vi "Host View Process.vi"(8 "error in (no error)":errorcluster, 11 "View Model":T8) -> (0 "error out":errorcluster)   [LabVIEW 2017]
doc: "PC Host based UI component for interaction with user"
uses:
  View Model/Controls/View Model.ctl
  View Model/Controls/Shared Model.ctl
  Error Handler/Controls/Error Model.ctl
  Error Handler/Controls/Error Event.ctl
  Error Handler/Controls/Error Type.ctl
  Controller/Controls/Controller Model.ctl
  Controller/Controls/Controller Event.ctl
  Controller/Controls/Controller Command.ctl
  Controller/Controls/Controller Overhead.ctl
  Real-Time/RT Status.ctl
  Real-Time/RT Loop Status.ctl
  Controller/Controls/Controller NStream.ctl
  Controller/Controls/Controller DAQ Data.ctl
  TDMS Logger/Controls/TDMS Model.ctl
  TDMS Logger/Controls/TDMS Event.ctl
  TDMS Logger/Controls/TDMS Command.ctl
  TDMS Logger/Controls/TDMS Overhead.ctl
  TDMS Logger/Controls/TDMS ChanProperties.ctl
  Controls/AIMV_GUI_Cluster.ctl
  Controls/AIMC_GUI_Cluster.ctl
  Controls/AOM_GUI_Cluster.ctl
  Controls/Discrete_GUI_Cluster.ctl
  Controls/GUI Referencies.ctl
  <resource>/objmgr/ni.dex.rc
panel:
  out "FileSize":i32
  out "Use TDMS?":bool
  in  "TDMS Close":bool
  in  "TDMS Save":bool
  in  "TDMS Create":bool
  in  "DOM7 Array":T1[](array[typedef])
  in  "DIM4 Array":T1[](array[typedef])
  out "DAQ Data":T2
  in  "DAQ read":bool
  in  "DAQ write":bool
  out "NStream.exist?":bool
  out "Available":i32
  out "size(s)":i32[](array[numeric])
  in  "NW Start/Stop":bool
  in  "DOM6 Array":T1[](array[typedef])
  in  "DIM3 Array":T1[](array[typedef])
  in  "AOM9 Array":T3[](array[typedef]) {"Ch.value" min=-10.0 max=20.0 step=1.0 format="%.3g"}
  in  "AIMC Array":T4[](array[typedef]) {"Ch.value" min=0.0 max=20.1 step=1.0 format="%.3g"}
  in  "AIM2 Array":T5[](array[typedef]) {"Ch.value" min=-10.0 max=10.0 step=1.0 format="%05.3f"}
  out "RT Status":T6 {"Status NPL"."Duration, us" format="%0.2f"; "Status TCL2"."Duration, us" format="%0.2f"; "Status TCL1"."Duration, us" format="%0.2f"}
  in  "Stop RT":bool
  out "Blink1":bool
  in  "Stop App":bool
  in  "Init":bool
  # "DAQ data"
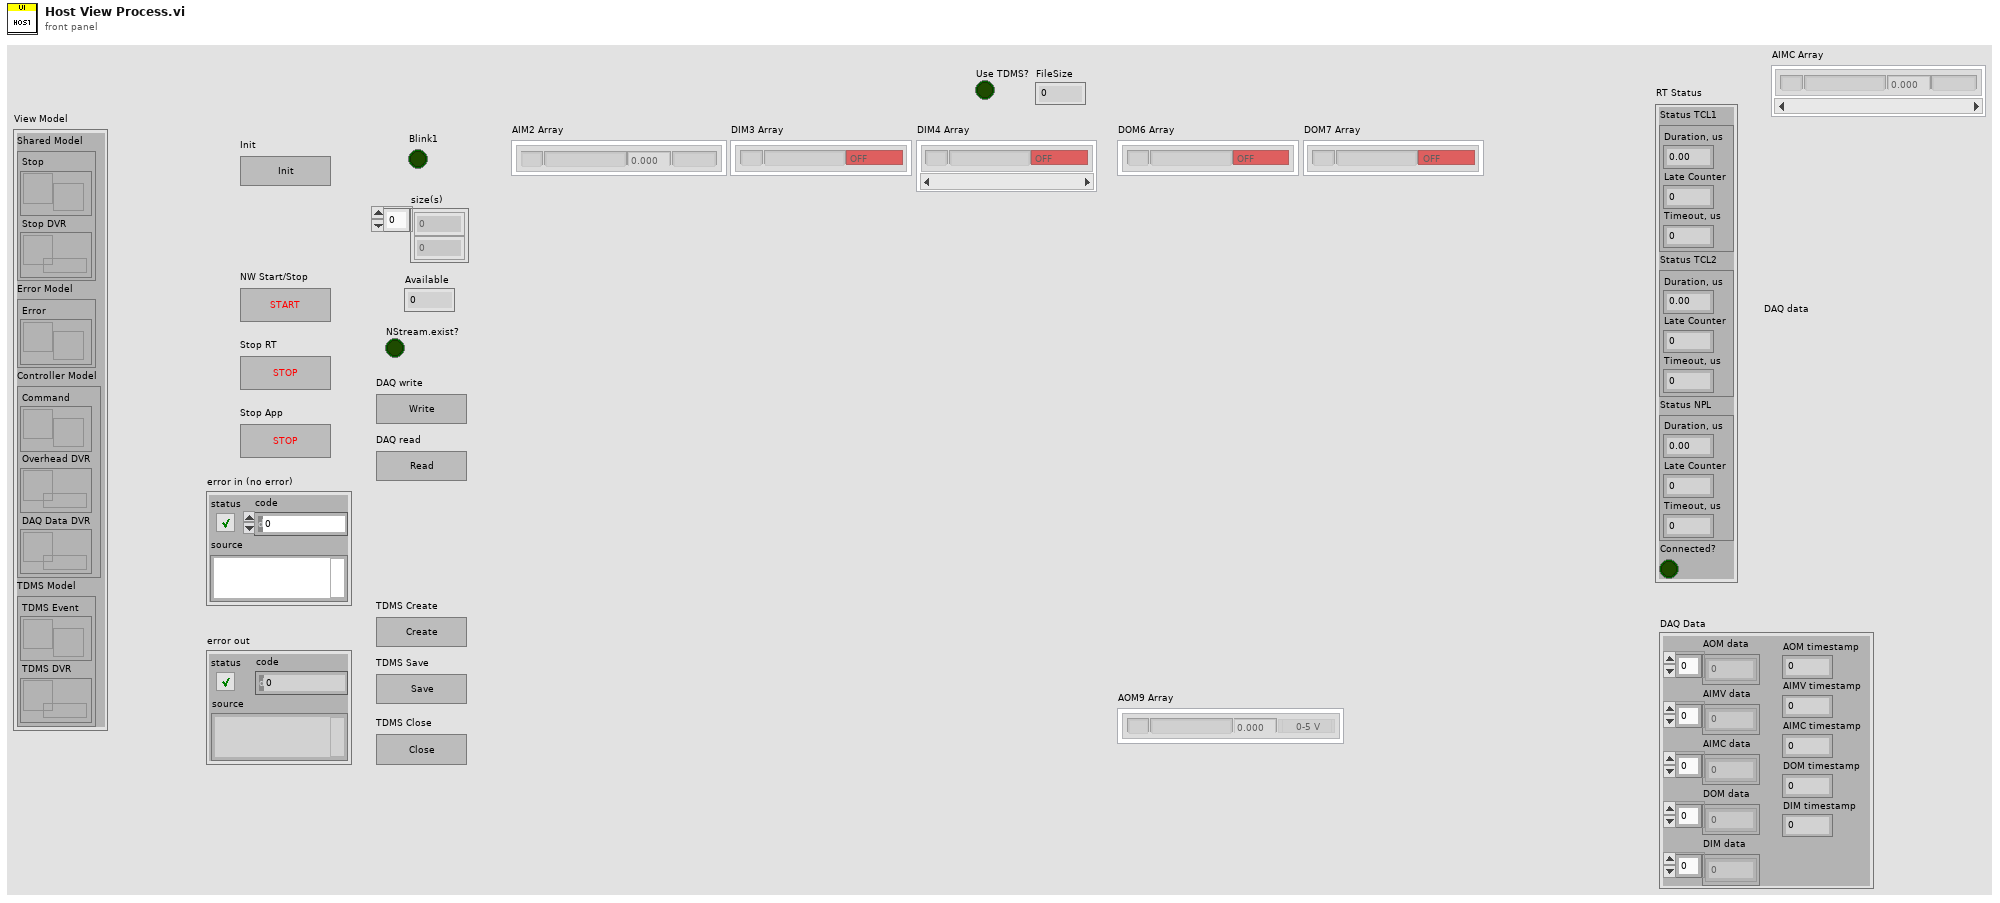
[diagram p1: front panel]
types:
  T1 = typedef "Discrete_GUI_Cluster.ctl" = cluster{"Ch.name":string, "Ch.state":bool, "Num":string}
  T2 = typedef "Controller DAQ Data.ctl" = cluster{"AOM data":dbl[], "AIMV data":dbl[], "AIMC data":dbl[], "DOM data":dbl[], "DIM data":dbl[], "AOM timestamp":dbl, "AIMV timestamp":dbl, "AIMC timestamp":dbl, "DOM timestamp":dbl, "DIM timestamp":dbl}
  T3 = typedef "AOM_GUI_Cluster.ctl" = cluster{"Ch.name":string, "Ch.value":dbl, "Ch.mode":enum16{"0-5 V", "+/-10 V", "0-5 mA", "4-20 mA"}, "Num":string}
  T4 = typedef "AIMC_GUI_Cluster.ctl" = cluster{"Ch.name":string, "Ch.value":dbl, "Ch.range":string, "Num":string}
  T5 = typedef "AIMV_GUI_Cluster.ctl" = cluster{"Ch.name":string, "Ch.value":dbl, "Ch.range":string, "Num":string}
  T6 = typedef "RT Status.ctl" = cluster{"Status TCL1":T7, "Status TCL2":T7, "Status NPL":T7, "Connected?":bool}
  T7 = typedef "RT Loop Status.ctl" = cluster{"Duration, us":dbl, "Late Counter":i32, "Timeout, us":u32}
  T8 = typedef "View Model.ctl" = cluster{"Shared Model":T9, "Error Model":T10, "Controller Model":T11, "TDMS Model":T12}
  T9 = typedef "Shared Model.ctl" = cluster{"Stop":refnum<user-event>, "Stop DVR":refnum<data-value>}
  T10 = typedef "Error Model.ctl" = cluster{"Error":refnum<user-event>}
  T11 = typedef "Controller Model.ctl" = cluster{"Command":refnum<user-event>, "Overhead DVR":refnum<data-value>, "DAQ Data DVR":refnum<data-value>}
  T12 = typedef "TDMS Model.ctl" = cluster{"TDMS Event":refnum<user-event>, "TDMS DVR":refnum<data-value>}
  T13 = typedef "GUI Referencies.ctl" = cluster{"This VI":refnum<vi>, "This App":refnum<vi>, "DIM3":refnum<vi>, "DIM4":refnum<vi>, "DOM6":refnum<vi>, "DOM7":refnum<vi>, "AOM9":refnum<vi>, "AIM2":refnum<vi>, "AIMC":refnum<vi>}
  T14 = typedef "Controller Command.ctl" = enum16{"Idle", "Init", "Stop App", "Stop RT", "NStream Create", "NStream Begin", "NStream End", "NStream Close", "DAQ Data Read", "DAQ Data Write", "TDMS Restart"}
  T15 = typedef "Error Type.ctl" = enum16{"Minor", "Critical"}
  T16 = typedef "TDMS Command.ctl" = enum16{"Idle", "Create File", "Save Data", "Close Fire"}
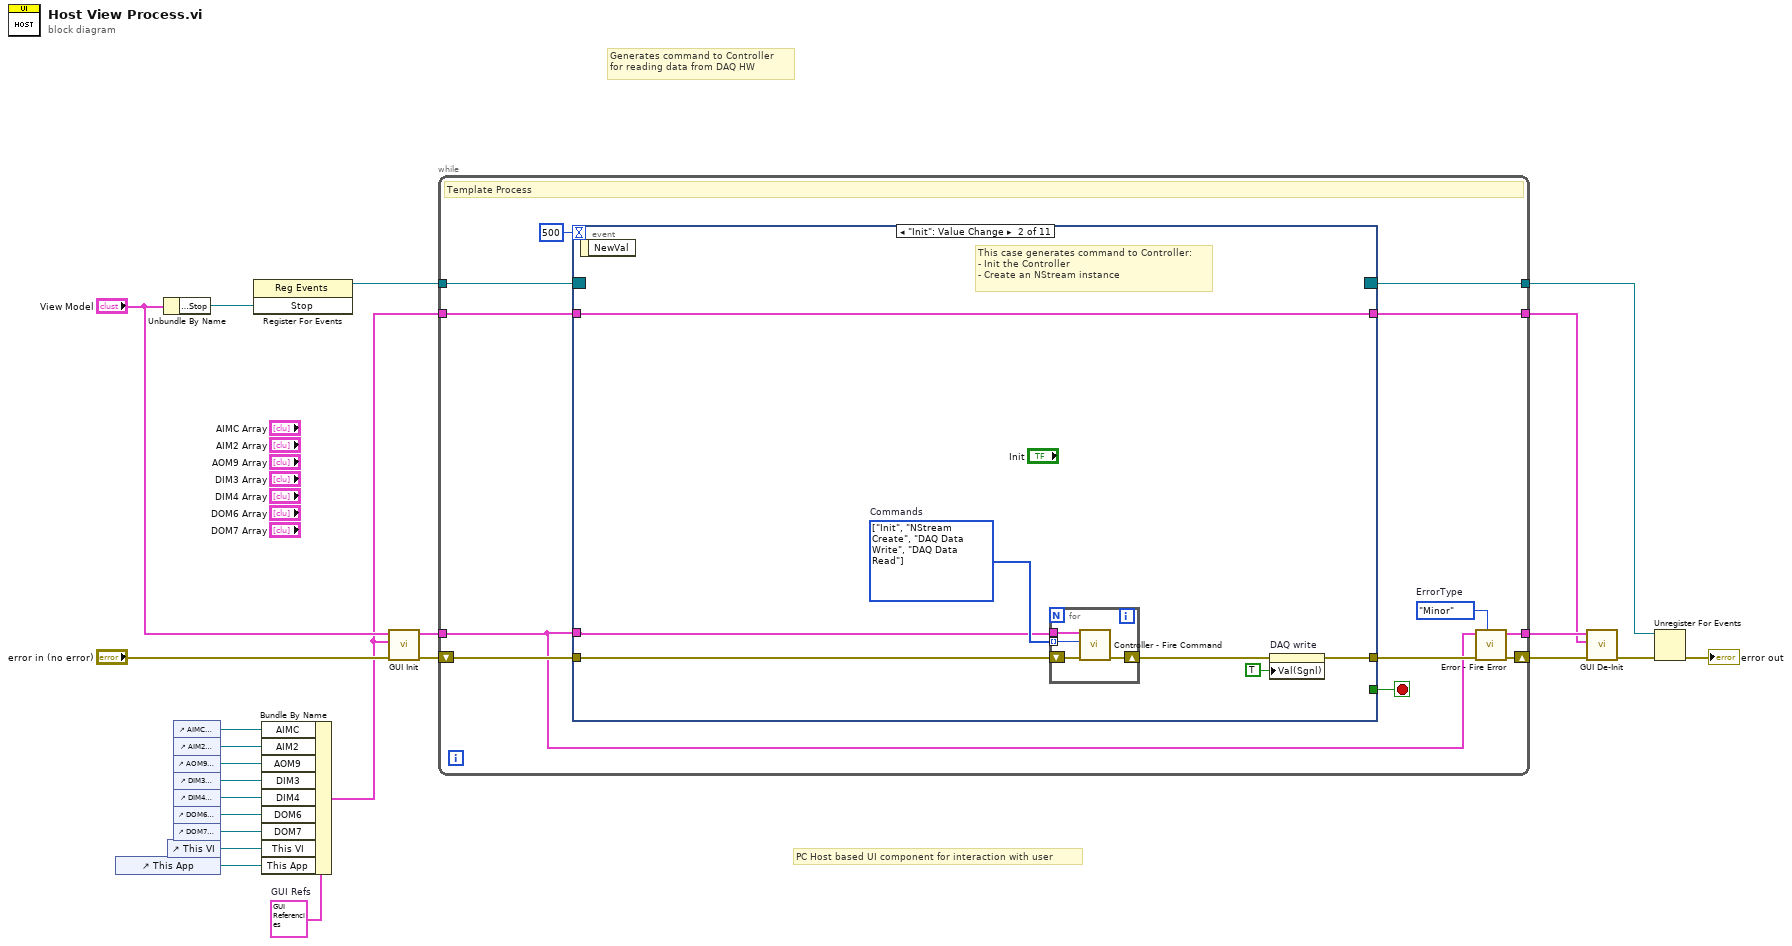
[diagram p0: block diagram]
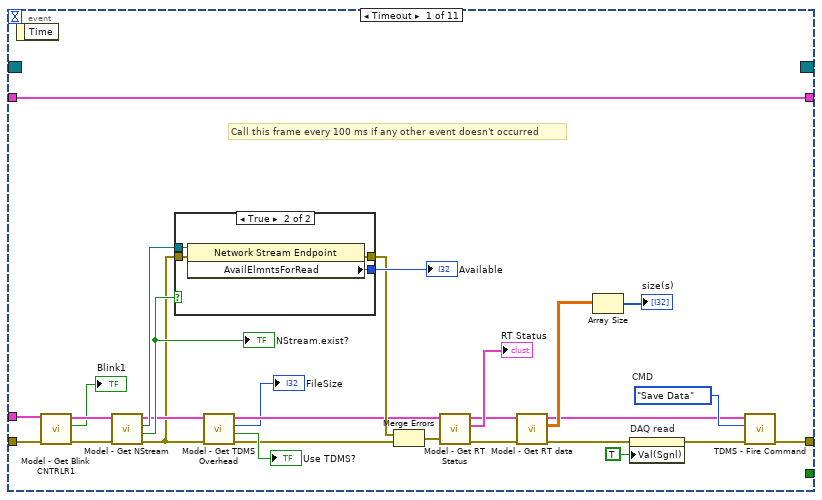
[diagram p2: hidden frame]
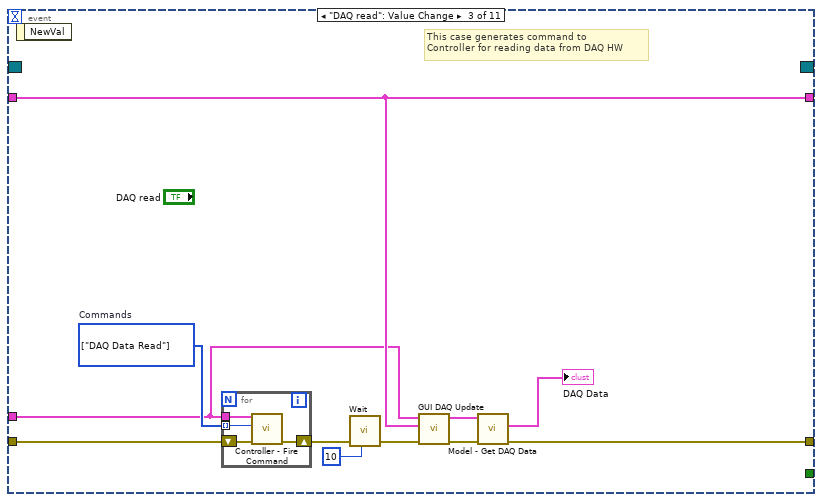
[diagram p4: hidden frame]
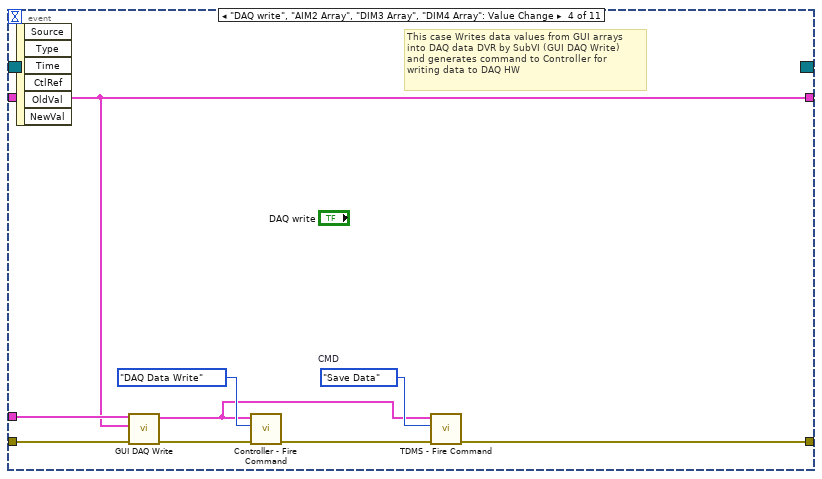
[diagram p5: hidden frame]
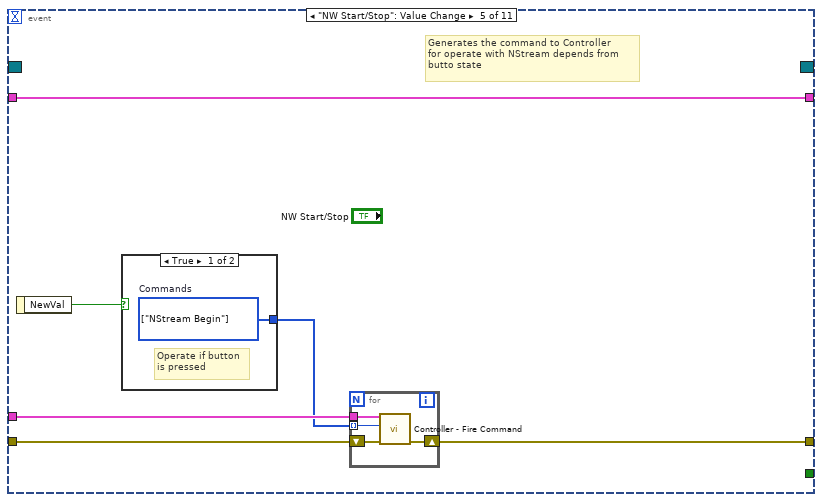
[diagram p6: hidden frame]
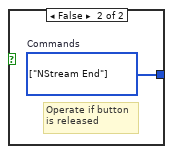
[diagram p7: hidden frame]
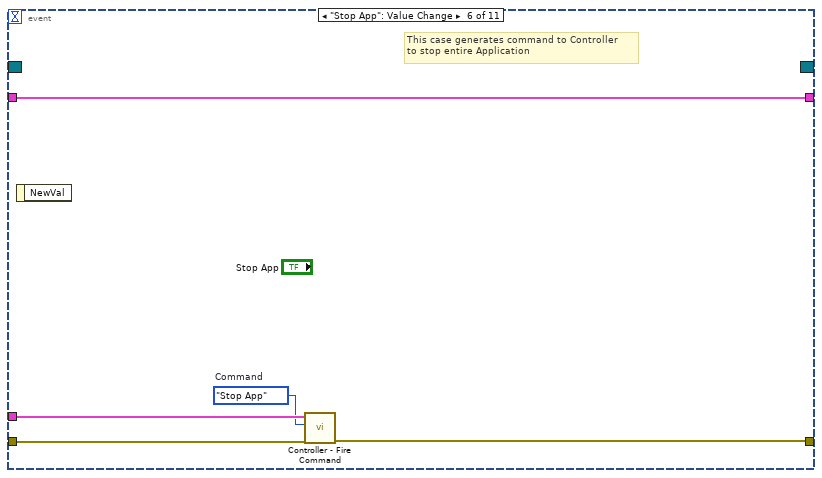
[diagram p8: hidden frame]
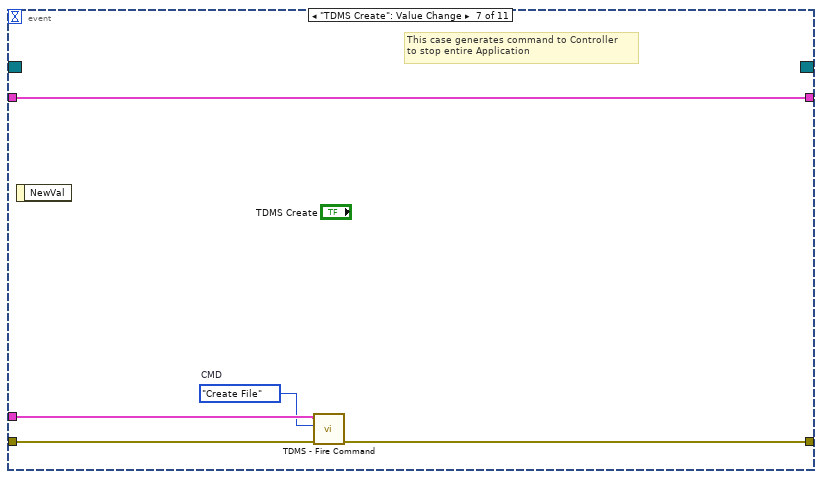
[diagram p9: hidden frame]
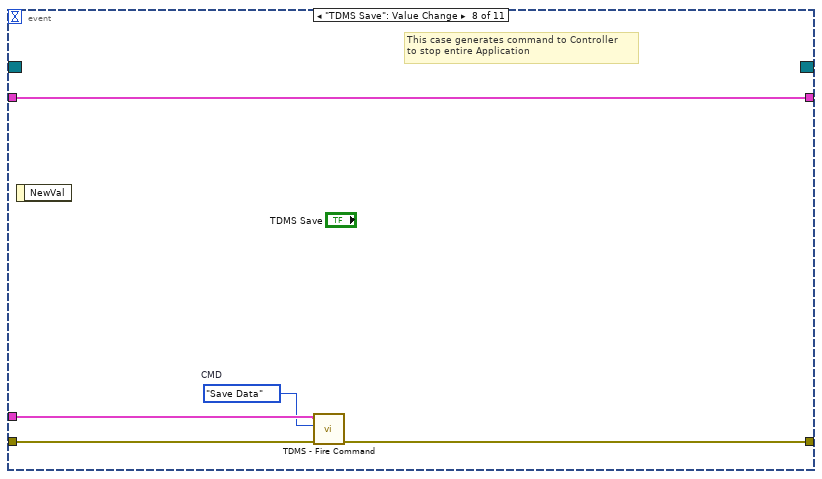
[diagram p10: hidden frame]
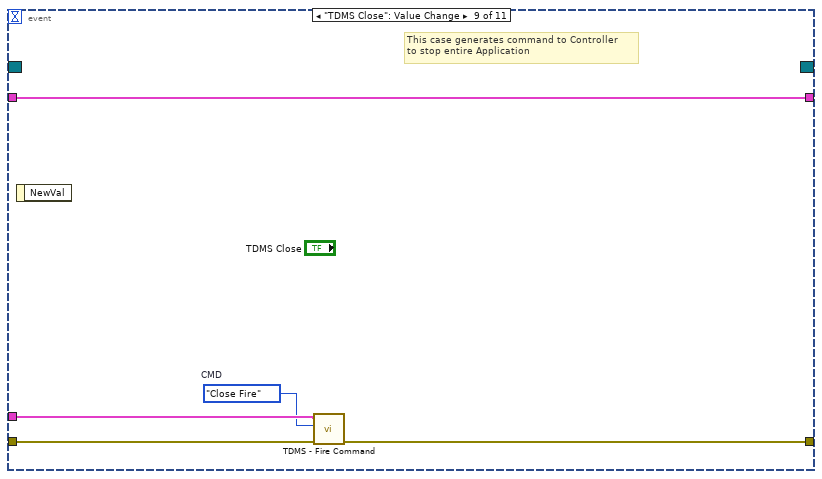
[diagram p11: hidden frame]
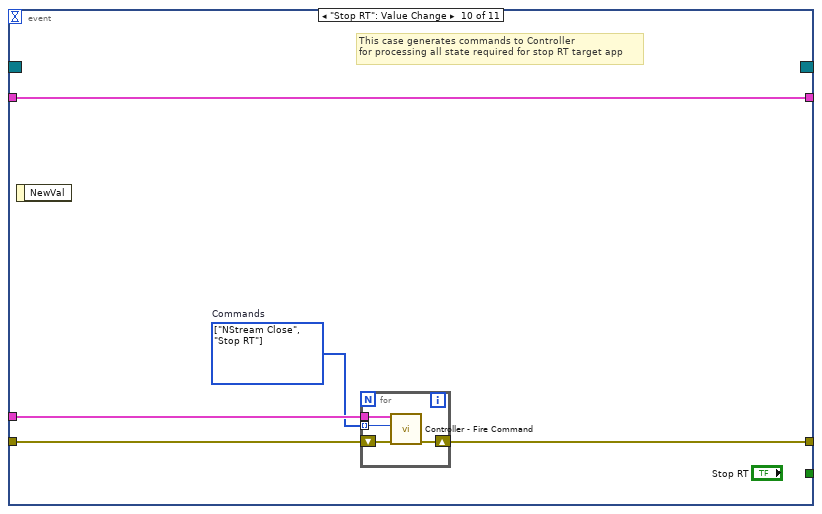
[diagram p12: hidden frame]
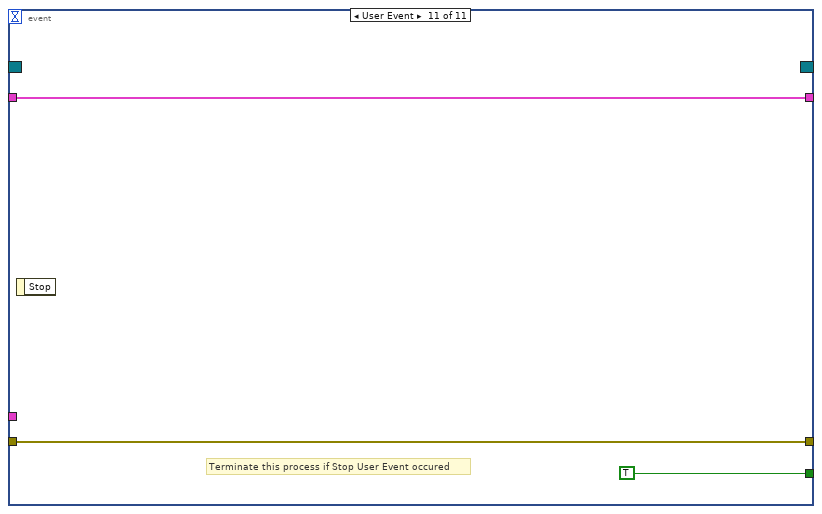
[diagram p13: hidden frame]
diagram:
  w12 = T13 {"This VI"=refnum, "This App"=refnum, "DIM3"=refnum, "DIM4"=refnum, "DOM6"=refnum, "DOM7"=refnum, "AOM9"=refnum, "AIM2"=refnum, "AIMC"=refnum}  # GUI Refs
  # "Generates command to Controller \nfor reading data from DAQ HW"
  # "PC Host based UI component for interaction with user"
  n1 = control-ref of="This App"() -> (w11:refnum<vi>)
  n2 = Unbundle By Name("View Model") -> ("Shared Model.Stop"=w23:refnum<user-event>)
  n3 = control-ref of="This VI"() -> (w10:refnum<vi>)
  n4 = control-ref of="AIMC Array"() -> (w1:refnum<vi>)
  n5 = control-ref of="AIM2 Array"() -> (w4:refnum<vi>)
  n6 = control-ref of="AOM9 Array"() -> (w3:refnum<vi>)
  n7 = control-ref of="DIM3 Array"() -> (w2:refnum<vi>)
  n8 = control-ref of="DIM4 Array"() -> (w5:refnum<vi>)
  n9 = control-ref of="DOM6 Array"() -> (w6:refnum<vi>)
  n10 = control-ref of="DOM7 Array"() -> (w7:refnum<vi>)
  n11 = register-events(w23) -> (reference out=w22:refnum<event-registration>)  [unwired: 2 in, 1 out]
  n12 = Bundle By Name(cluster=w12, "AIMC"=w1, "AIM2"=w4, "AOM9"=w3, "DIM3"=w2, "DIM4"=w5, "DOM6"=w6, "DOM7"=w7, "This VI"=w10, "This App"=w11) -> (w9:T13)
  n13 = call "GUI Init.vi"("error in (no error)"="error in (no error)", "GUI Refs"=w9, "View Model"="View Model") -> ("error out"=w18:errorcluster, "View Model"=w16:T8)  [unwired: 7 in]
  n14 = while {
    tunnel: w22 -> [w33]
    shift-right: [w29] -> w15
    shift-left: w18 -> [w35]
    tunnel: w16 -> [w28]
    tunnel: [w32] -> w21
    tunnel: [w27] -> w14
    tunnel: w9 -> [w25]
    tunnel: [w24] -> w8
    stop <- w31 stop-if-true
    w26 = Error_Type."Minor"  # ErrorType
    # "Template Process"
    n15 = event shown="[1] \"Init\": Value Change" {
      selector: w33 -> [_ _ _ _ _ _ _ _ _ _ _]
      dyn-events: [_ _ _ _ _ _ _ _ _ _ _] -> w32
      timeout: 500 -> [_ _ _ _ _ _ _ _ _ _ _]
      tunnel: w35 -> [w63 w69 w90 w103 w109 w120 w124 w129 w134 w140 w147]
      tunnel: w28 -> [w62 w70 w81 w102 w108 w119 w122 w127 w132 w139 _]
      tunnel: [w46 w72 w83 w96 w107 w118 w123 w128 w133 w138 w147] -> w30
      tunnel: [_ _ _ _ _ _ _ _ _ _ TRUE] -> w31
      tunnel: w25 -> [w51 w74 w82 w101 w104 w116 w125 w130 w135 w136 w145]
      tunnel: [w51 w74 w82 w101 w104 w116 w125 w130 w135 w136 w145] -> w24
      event Timeout {
        w48 = TDMS_Command."Save Data"  # CMD
        # "Call this frame every 100 ms if any other event doesn't occurred"
        n16 = event-data() -> ()  [unwired: 1 in, 1 out]
        n17 = call "Model - Get Blink CNTRLR1.vi"("error in (no error)"=w63, "View Model"=w62) -> ("error out"=w55:errorcluster, "BlinkC1"=→"Blink1":bool, "View Model"=w56:T8)  [unwired: 7 in]
        n18 = call "Model - Get NStream.vi"("error in (no error)"=w55, "View Model"=w56) -> ("error out"=w44:errorcluster, "NStream.exist?"=w52:bool, "NStream.Endpoint"=w54:refnum<k21>, "View Model"=w45:T8)  [unwired: 6 in]
        "NStream.exist?" <- w52
        n19 = case shown="True" w52 {
          tunnel: w44 -> [w64 w68]
          tunnel: w54 -> [_ w67]
          tunnel: [w64 w66] -> w49
          tunnel: [_ w65] -> w53
          frame False {
          }
          frame True {
            n20 = property class="Network Stream Endpoint"(reference=w67, error in=w68) -> (error out=w66:errorcluster, "AvailElmntsForRead"=w65:i32)  [unwired: 1 out]
          }
        }
        "Available" <- w53
        n21 = call "Model - Get TDMS Overhead.vi"("error in (no error)"=w44, "View Model"=w45) -> ("error out"=w40:errorcluster, "Use TDMS?"=→"Use TDMS?":bool, "FileSize"=→"FileSize":i32, "View Model"=w43:T8)  [unwired: 4 in, 2 out]
        n22 = Merge Errors(w49, w40) -> (w50:errorcluster)
        n23 = call "Model - Get RT Status.vi"("error in (no error)"=w50, "View Model"=w43) -> ("error out"=w60:errorcluster, "RT Status"=→"RT Status":T6, "View Model"=w59:T8)  [unwired: 7 in]
        n24 = call "Model - Get RT data.vi"("error in (no error)"=w60, "View Model"=w59) -> ("error out"=w39:errorcluster, "RT data"=w58:dbl[][], "View Model"=w47:T8)  [unwired: 7 in]
        n25 = Array Size(array=w58) -> (size(s)=→"size(s)":i32[])
        n26 = property on="DAQ read" class="Bool (strict)"(error in=w39, "Val(Sgnl)"=TRUE ("Value (Signaling)")) -> (error out=w38:errorcluster)  [unwired: 1 in, 1 out]
        n27 = call "TDMS - Fire Command.vi"("error in (no error)"=w38, "CMD"=w48, "View Model"=w47) -> ("error out"=w46:errorcluster)  [unwired: 8 in]
      }
      event "Init": Value Change {
        w75 = T14[] [enum."Init", enum."NStream Create", enum."DAQ Data Write", enum."DAQ Data Read"] items=["Idle", "Init", "Stop App", "Stop RT", "NStream Create", "NStream Begin", "NStream End", "NStream Close", "DAQ Data Read", "DAQ Data Write", "TDMS Restart"]  # Commands
        # "This case generates command to Controller:\n- Init the Controller\n- Create an NStream instance"
        n28 = event-data() -> ()  [unwired: 1 in, 1 out]
        n29 = for {
          tunnel: w70 -> [w78]
          shift-right: [w77] -> w73
          shift-left: w69 -> [w79]
          tunnel: w75 -> [w76] mode=indexing
          n30 = call "Controller - Fire Command.vi"("error in (no error)"=w79, "CMD"=w76, "View Model"=w78) -> ("error out"=w77:errorcluster)  [unwired: 8 in]
        }
        n31 = property on="DAQ write" class="Bool (strict)"(error in=w73, "Val(Sgnl)"=TRUE ("Value (Signaling)")) -> (error out=w72:errorcluster)  [unwired: 1 in, 1 out]
      }
      event "DAQ read": Value Change {
        w89 = T14[] [enum."DAQ Data Read"] items=["Idle", "Init", "Stop App", "Stop RT", "NStream Create", "NStream Begin", "NStream End", "NStream Close", "DAQ Data Read", "DAQ Data Write", "TDMS Restart"]  # Commands
        # "This case generates command to \nController for reading data from DAQ HW"
        n32 = event-data() -> ()  [unwired: 1 in, 1 out]
        n33 = for {
          tunnel: w81 -> [w93]
          shift-right: [w92] -> w88
          shift-left: w90 -> [w94]
          tunnel: w89 -> [w91] mode=indexing
          n34 = call "Controller - Fire Command.vi"("error in (no error)"=w94, "CMD"=w91, "View Model"=w93) -> ("error out"=w92:errorcluster)  [unwired: 8 in]
        }
        n35 = call "Wait.vi"("error in (no error)"=w88, "wait, ms"=u32 10) -> ("error out"=w84:errorcluster)  [unwired: 7 in]
        n36 = call "GUI DAQ Update.vi"("error in (no error)"=w84, "GUI Refs"=w82, "View Model"=w81) -> ("error out"=w86:errorcluster, "View Model"=w85:T8)  [unwired: 7 in]
        n37 = call "Model - Get DAQ Data.vi"("error in (no error)"=w86, "View Model"=w85) -> ("error out"=w83:errorcluster, "DAQ Data"=→"DAQ Data":T2)  [unwired: 7 in, 1 out]
      }
      event "DAQ write", "AIM2 Array", "DIM3 Array", "DIM4 Array": Value Change {
        w98 = TDMS_Command."Save Data"  # CMD
        # "This case Writes data values from GUI arrays\ninto DAQ data DVR by SubVI (GUI DAQ Write)\nand generates command to Controller for \nwriting data to DAQ HW"
        n38 = event-data() -> ()  [unwired: 1 in, 6 out]
        n39 = call "GUI DAQ Write.vi"("error in (no error)"=w103, "GUI Refs"=w101, "View Model"=w102) -> ("error out"=w100:errorcluster, "View Model"=w95:T8)  [unwired: 7 in]
        n40 = call "Controller - Fire Command.vi"("error in (no error)"=w100, "CMD"=Controller_Command."DAQ Data Write", "View Model"=w95) -> ("error out"=w97:errorcluster)  [unwired: 8 in]
        n41 = call "TDMS - Fire Command.vi"("error in (no error)"=w97, "CMD"=w98, "View Model"=w95) -> ("error out"=w96:errorcluster)  [unwired: 8 in]
      }
      event "NW Start/Stop": Value Change {
        # "Generates the command to Controller\nfor operate with NStream depends from\nbutto state"
        n42 = event-data() -> ("NewVal"=w106:bool)  [unwired: 1 in]
        n43 = case shown="True" w106 {
          tunnel: [w110 w111] -> w105
          frame True {
            w110 = T14[] [enum."NStream Begin"] items=["Idle", "Init", "Stop App", "Stop RT", "NStream Create", "NStream Begin", "NStream End", "NStream Close", "DAQ Data Read", "DAQ Data Write", "TDMS Restart"]  # Commands
            # "Operate if button\nis pressed"
          }
          frame False {
            w111 = T14[] [enum."NStream End"] items=["Idle", "Init", "Stop App", "Stop RT", "NStream Create", "NStream Begin", "NStream End", "NStream Close", "DAQ Data Read", "DAQ Data Write", "TDMS Restart"]  # Commands
            # "Operate if button\nis released"
          }
        }
        n44 = for {
          tunnel: w108 -> [w114]
          shift-right: [w113] -> w107
          shift-left: w109 -> [w115]
          tunnel: w105 -> [w112] mode=indexing
          n45 = call "Controller - Fire Command.vi"("error in (no error)"=w115, "CMD"=w112, "View Model"=w114) -> ("error out"=w113:errorcluster)  [unwired: 8 in]
        }
      }
      event "Stop App": Value Change {
        w117 = Controller_Command."Stop App"  # Command
        # "This case generates command to Controller\nto stop entire Application"
        n46 = event-data() -> ()  [unwired: 1 in, 1 out]
        n47 = call "Controller - Fire Command.vi"("error in (no error)"=w120, "CMD"=w117, "View Model"=w119) -> ("error out"=w118:errorcluster)  [unwired: 8 in]
      }
      event "TDMS Create": Value Change {
        w121 = TDMS_Command."Create File"  # CMD
        # "This case generates command to Controller\nto stop entire Application"
        n48 = event-data() -> ()  [unwired: 1 in, 1 out]
        n49 = call "TDMS - Fire Command.vi"("error in (no error)"=w124, "CMD"=w121, "View Model"=w122) -> ("error out"=w123:errorcluster)  [unwired: 8 in]
      }
      event "TDMS Save": Value Change {
        w126 = TDMS_Command."Save Data"  # CMD
        # "This case generates command to Controller\nto stop entire Application"
        n50 = event-data() -> ()  [unwired: 1 in, 1 out]
        n51 = call "TDMS - Fire Command.vi"("error in (no error)"=w129, "CMD"=w126, "View Model"=w127) -> ("error out"=w128:errorcluster)  [unwired: 8 in]
      }
      event "TDMS Close": Value Change {
        w131 = TDMS_Command."Close Fire"  # CMD
        # "This case generates command to Controller\nto stop entire Application"
        n52 = event-data() -> ()  [unwired: 1 in, 1 out]
        n53 = call "TDMS - Fire Command.vi"("error in (no error)"=w134, "CMD"=w131, "View Model"=w132) -> ("error out"=w133:errorcluster)  [unwired: 8 in]
      }
      event "Stop RT": Value Change {
        w137 = T14[] [enum."NStream Close", enum."Stop RT"] items=["Idle", "Init", "Stop App", "Stop RT", "NStream Create", "NStream Begin", "NStream End", "NStream Close", "DAQ Data Read", "DAQ Data Write", "TDMS Restart"]  # Commands
        # "This case generates commands to Controller\nfor processing all state required for stop RT target app"
        n54 = event-data() -> ()  [unwired: 1 in, 1 out]
        n55 = for {
          tunnel: w139 -> [w143]
          shift-right: [w142] -> w138
          shift-left: w140 -> [w144]
          tunnel: w137 -> [w141] mode=indexing
          n56 = call "Controller - Fire Command.vi"("error in (no error)"=w144, "CMD"=w141, "View Model"=w143) -> ("error out"=w142:errorcluster)  [unwired: 8 in]
        }
      }
      event User Event {
        # "Terminate this process if Stop User Event occured"
        n57 = event-data() -> ()  [unwired: 1 in, 1 out]
      }
    }
    n58 = call "Error - Fire Error.vi"("ErrorType"=w26, "error in (no error)"=w30, "View Model"=w28) -> ("error out"=w29:errorcluster, "View Model"=w27:T8)  [unwired: 7 in]
  }
  n59 = call "GUI De-Init.vi"("error in (no error)"=w15, "GUI Refs"=w8, "View Model"=w14) -> ("error out"=w13:errorcluster)  [unwired: 7 in, 1 out]
  n60 = Unregister For Events(event registration refnum=w21, error in=w13) -> (error out=→"error out":errorcluster)
